vi "DeleteData.vi"(8 "error in (no error)":errorcluster, 10 "Select Conditions Criteria":T1, 11 "object in":refnum<class "TableLogger_SQLite_Actor.lvclass">) -> (0 "error out":errorcluster, 2 "Data Clusters":variant[](array[variant]), 3 "object out":refnum<class "TableLogger_SQLite_Actor.lvclass">)   [LabVIEW 2014, in "TableLogger_SQLite_Actor.lvlib" / "TableLogger_SQLite_Actor.lvclass"]
uses:
  TableLogger_SQLite_Actor.lvclass
  TableLogger_Actor/SelectConditionCriteria.ctl
  SelectConditions.ctl
  TableLogger_SQLite_Actor.lvclass/TableLogger_SQLite_Actor.ctl
  <vilib>/drjdpowell/SQLite Library/SQL Connection/Execute SQL.vi
  <vilib>/drjdpowell/SQLite Library/SQLite.lvlib
  <vilib>/drjdpowell/SQLite Library/SQL Connection/Connection.lvclass
  TableLogger_Actor/TableLogger_Actor/TableLogger_Actor.lvclass
  TableLogger_Actor/TableLogger_Actor.lvlib
panel:
  # "Connector Pane"
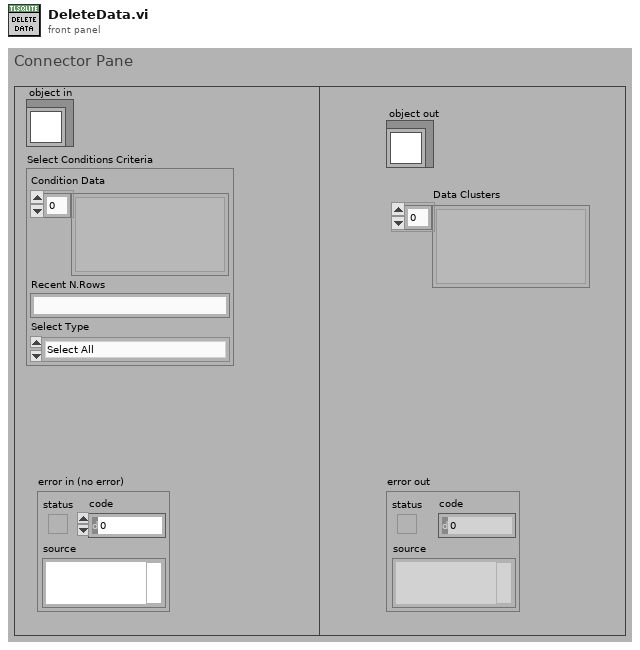
[diagram p1: front panel]
types:
  T1 = typedef "TableLogger_Actor.lvlib/SelectConditionCriteria.ctl" = cluster{"Condition Data":variant[], "Recent N.Rows":string, "Select Type":T2}
  T2 = typedef "TableLogger_Actor.lvlib/SelectConditions.ctl" = enum16{"Select All", "AND Operator", "Recent Rows", "OR Operator", "BETWEEN Operator"}
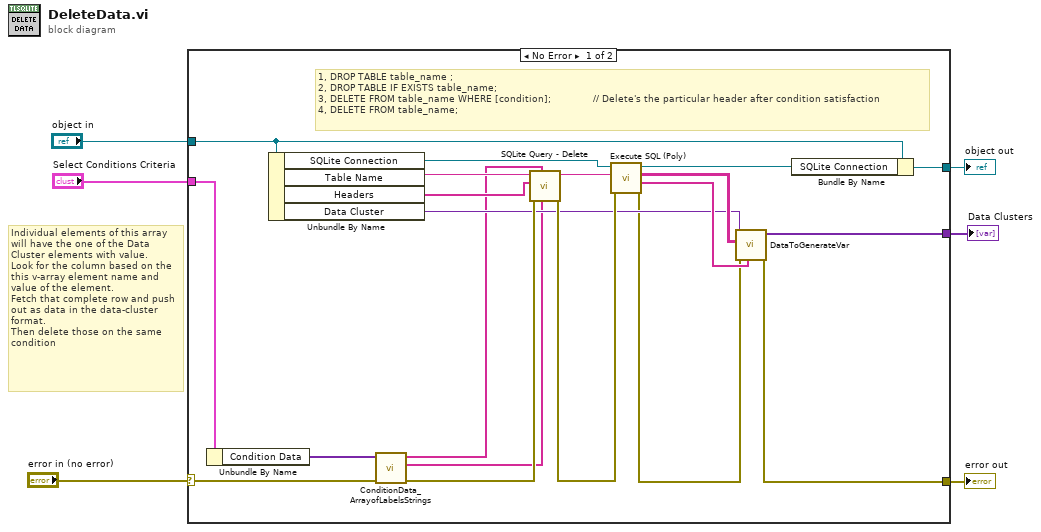
[diagram p0: block diagram]
diagram:
  # "Individual elements of this array will have the one of the Data Cluster elements with value.\nLook for the column based on the this v-array element name and value of the element.\nFetch that complete row and push out as data in the data-cluster format.\nThen delete those on the same condition"
  n1 = case shown="No Error" "error in (no error)" {
    selector: "error in (no error)" -> [w18 w28]
    tunnel: [w11 w28] -> w5
    tunnel: [w26 w27] -> w3
    tunnel: "object in" -> [w25 w27]
    tunnel: "Select Conditions Criteria" -> [w16 _]
    tunnel: [w10 _] -> w2
    frame No Error {
      # "1, DROP TABLE table_name ;\n2, DROP TABLE IF EXISTS table_name;\n3, DELETE FROM table_name WHERE [condition];              // Delete's the particular header after condition satisfaction\n4, DELETE FROM table_name;"
      n2 = Unbundle By Name(w16) -> ("Condition Data"=w7:variant[])
      n3 = Unbundle By Name(w25) -> ("SQLite Connection"=w23:refnum<class "Connection.lvclass">, "Table Name"=w22:string, "Headers"=w19:string[], "Data Cluster"=w13:variant)
      n4 = call "ConditionData_ArrayofLabelsStrings.vi"("error in (no error)"=w18, "Condition Data"=w7) -> ("error out"=w17:errorcluster, "Value"=w8:string[], "Label"=w9:string[])  [unwired: 7 in]
      n5 = call "SQLite Query - Delete.vi"("A[Strings] Value"=w8, "A[Strings]"=w9, "error in"=w17, "Table Headers"=w19, "Table Name"=w22) -> ("error out"=w20:errorcluster, "SQLite Query"=w21:string)  [unwired: 5 in]
      n6 = call-poly <vilib>:"Execute SQL (Poly).vi"("error in (no error)"=w20, "SQL"=w21, "SQLite Connection in"=w23) -> ("error out"=w12:errorcluster, "Column Names"=w14:string[], "Result Set"=w15:string[][], "SQLite Connection"=w24:refnum<class "Connection.lvclass">)  [unwired: 5 in]
      n7 = call "DataToGenerateVar.vi"("Header"=w14, "error in (no error)"=w12, "Data in"=w15, "Variant"=w13) -> ("error out"=w11:errorcluster, "Data"=w10:variant[])  [unwired: 6 in]
      n8 = Bundle By Name(cluster=w25, "SQLite Connection"=w24) -> (w26:refnum<class "TableLogger_SQLite_Actor.lvclass">)
    }
    frame Error {
    }
  }
  "error out" <- w5
  "object out" <- w3
  "Data Clusters" <- w2
